vi "Read Multi Boolean.vi"(8 "error in (no error)":errorcluster, 9 "Type":bool[](array[boolean]), 10 "Tags":string[](array[string]), 11 "Var Bus in":refnum<class "Omni_Bus.lvclass">) -> (0 "error out":errorcluster, 2 "Booleans":bool[](array[boolean]), 3 "Var Bus out":refnum<class "Omni_Bus.lvclass">)   [LabVIEW 2021, in "Omni_Bus.lvclass"]
uses:
  Omni_Bus.lvclass
  <vilib>/TSA/Abstract Data Classes/Abs_Types/Boolean/Abs_Boolean.lvclass
  Omni_Bus.lvclass/Omni_Bus.ctl
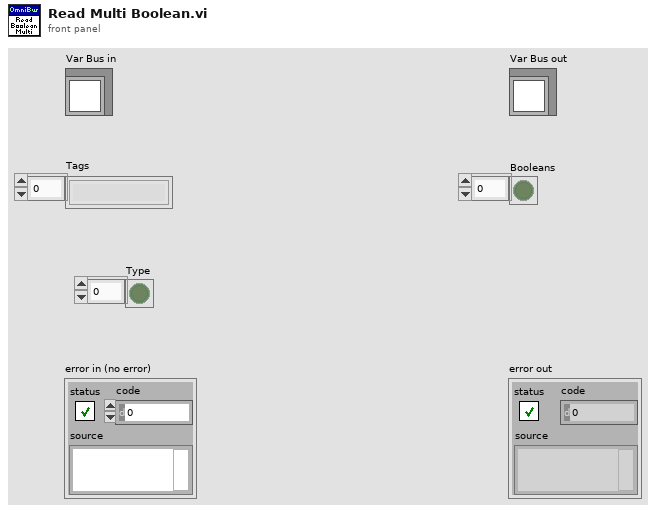
[diagram p1: front panel]
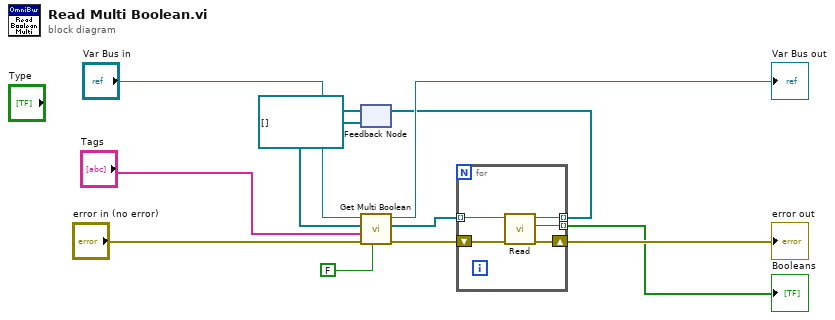
[diagram p0: block diagram]
diagram:
  n1 = feedback #1(refnum<class "Abs_Boolean.lvclass">[] []) -> (w8:refnum<class "Abs_Boolean.lvclass">[])
  n2 = call-dynamic "Get Multi Boolean.vi"("Write?"=FALSE, "error in (no error)"="error in (no error)", "Tag"="Tags", "Value Type"=w8, "Var Bus in"="Var Bus in") -> ("error out"=w7:errorcluster, "Value Out"=w6:refnum<class "Abs_Boolean.lvclass">[], "Var Bus out"=→"Var Bus out":refnum<class "Omni_Bus.lvclass">)  [unwired: 4 in]
  n3 = for {
    tunnel: w6 -> [w16] mode=indexing
    tunnel: [w14] -> w4 mode=indexing
    tunnel: [w13] -> w3 mode=indexing
    shift-right: [w15] -> w5
    shift-left: w7 -> [w17]
    n4 = call-dynamic "Read.vi"("error in (no error)"=w17, "Boolean in"=w16) -> ("error out"=w15:errorcluster, "Boolean"=w13:bool, "Boolean out"=w14:refnum<class "Abs_Boolean.lvclass">)  [unwired: 7 in]
  }
  "error out" <- w5
  "Booleans" <- w3
  n5 = feedback-in #1(w4) -> ()
